vi "interfaz.vi"() -> ()   [LabVIEW 2020]
uses:
  proceso2.vi
  proceso1.vi
  proceso3.vi
  proceso5.vi
  proceso6.vi
  proceso4.vi
panel:
  in  "stop":bool
  out "TEMPERATURA  FINAL":dbl
  out "TEMPERATURA REFIRGERADOR":dbl
  out "caja 2":u8(slide) scale=0.0..100.0
  out "vent3":bool
  out "vent2":bool
  out "vent1":bool
  out "CONTADOR DE CAJAS":dbl
  out "sensor_caja":bool
  out "TEMPERATURA  INTERCAMBIADOR":dbl
  out "caja":u8(slide) scale=0.0..100.0
  out "sensor_inter":bool
  out "sensor_final":bool
  out "tuberia_5":u8(slide) scale=0.0..100.0
  out "tuberia_3":u8(slide) scale=0.0..100.0
  out "tuberia_6":u8(slide) scale=0.0..100.0
  out "tuberia_2":u8(slide) scale=0.0..100.0
  out "tuberia_4":u8(slide) scale=0.0..100.0
  out "tuberia_1":u8(slide) scale=0.0..100.0
  out "tanque_out":u8(slide) scale=0.0..100.0
  out "tanque in":u8(slide) scale=0.0..100.0
  out "sensor_ref":bool
  out "sensor bomba 1":bool
  out "sensor bomba dos":bool
  out "sensor_cal":bool
  # "SISTEMA DE PASTEURIZACION DE LECHE"
  # "TANQUE DE ENTRADA"
  # "TANQUE OUT"
  # "FINAL DE LINEA"
  # "DISTRIBUIDORA"
  # "REFRIGERADOR"
  # "INTERCAMBIADOR DE CALOR"
  # "BOMBA 1"
  # "CALDERA"
  # "BOMBA 2"
  # "PANEL"
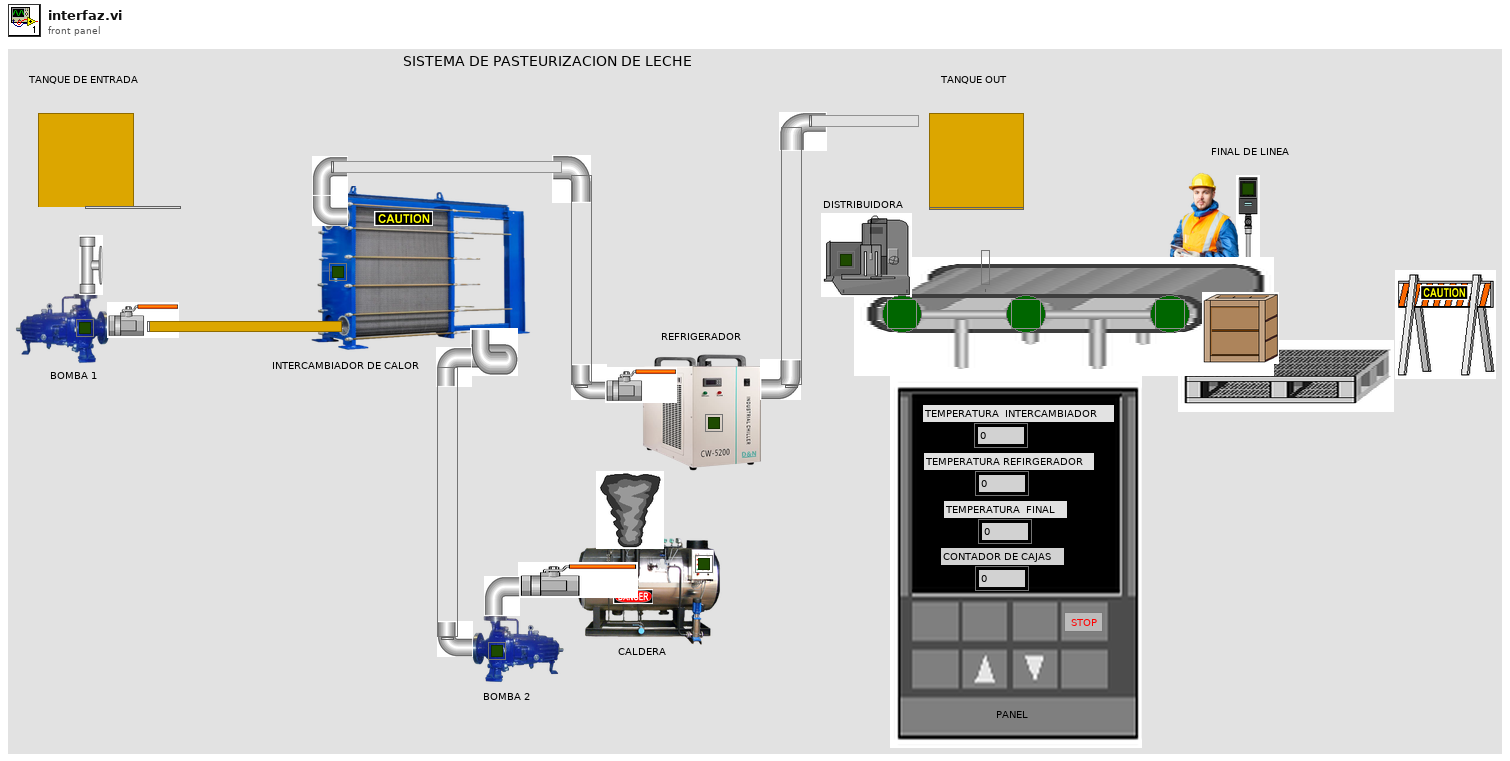
[diagram p1: front panel]
types:
  T1 = cluster{"final_linea":bool, "vent 1":bool, "vent 2":bool, "vent 3":bool, "mov caja horizontal":i32, "llenado caja":u8, "pos_inicial_horizontal":dbl, " pos_final_horizontal":dbl, "contador":dbl, "mov caja  vertical":i32, "pos_inicial_vertical":dbl, " pos_final_vertical":dbl}
  T2 = cluster{"sensor_caja":bool, "vent 1":bool, "vent 2":bool, "vent 3":bool, "pos_inicial":dbl, "pos_final":dbl, "mov_caja":i32}
  T3 = cluster{"sensor_refrigerador":bool, "temperatura":dbl, "tuberia 5":u8, "tuberia 6":u8}
  T4 = cluster{"sensor_bomba_1":bool, "tanque in":u8, " tuberia 1":u8}
  T5 = cluster{"sensor_intercambiador":bool, "sensor_caldera":bool, "sensor_bomba_2 ":bool, "tuberia 2":u8, "tuberia 3":u8, "tuberia 4":u8, "temperatura":dbl}
  T6 = cluster{"sensor_caja":bool, "vent 1":bool, "vent 2":bool, "vent 3":bool, "pos_inicial":dbl, "pos_final":dbl, "mov_caja 1":i32}
  T7 = cluster{"final_linea":bool, "vent 1":bool, "vent 2":bool, "vent 3":bool, "mov caja 2 horizontal":i32, "llenado caja 2":u8, "pos_inicial_horizontal":dbl, " pos_final_horizontal":dbl, "contador":dbl, "mov caja 2  vertical":i32, "pos_inicial_vertical":dbl, " pos_final_vertical":dbl}
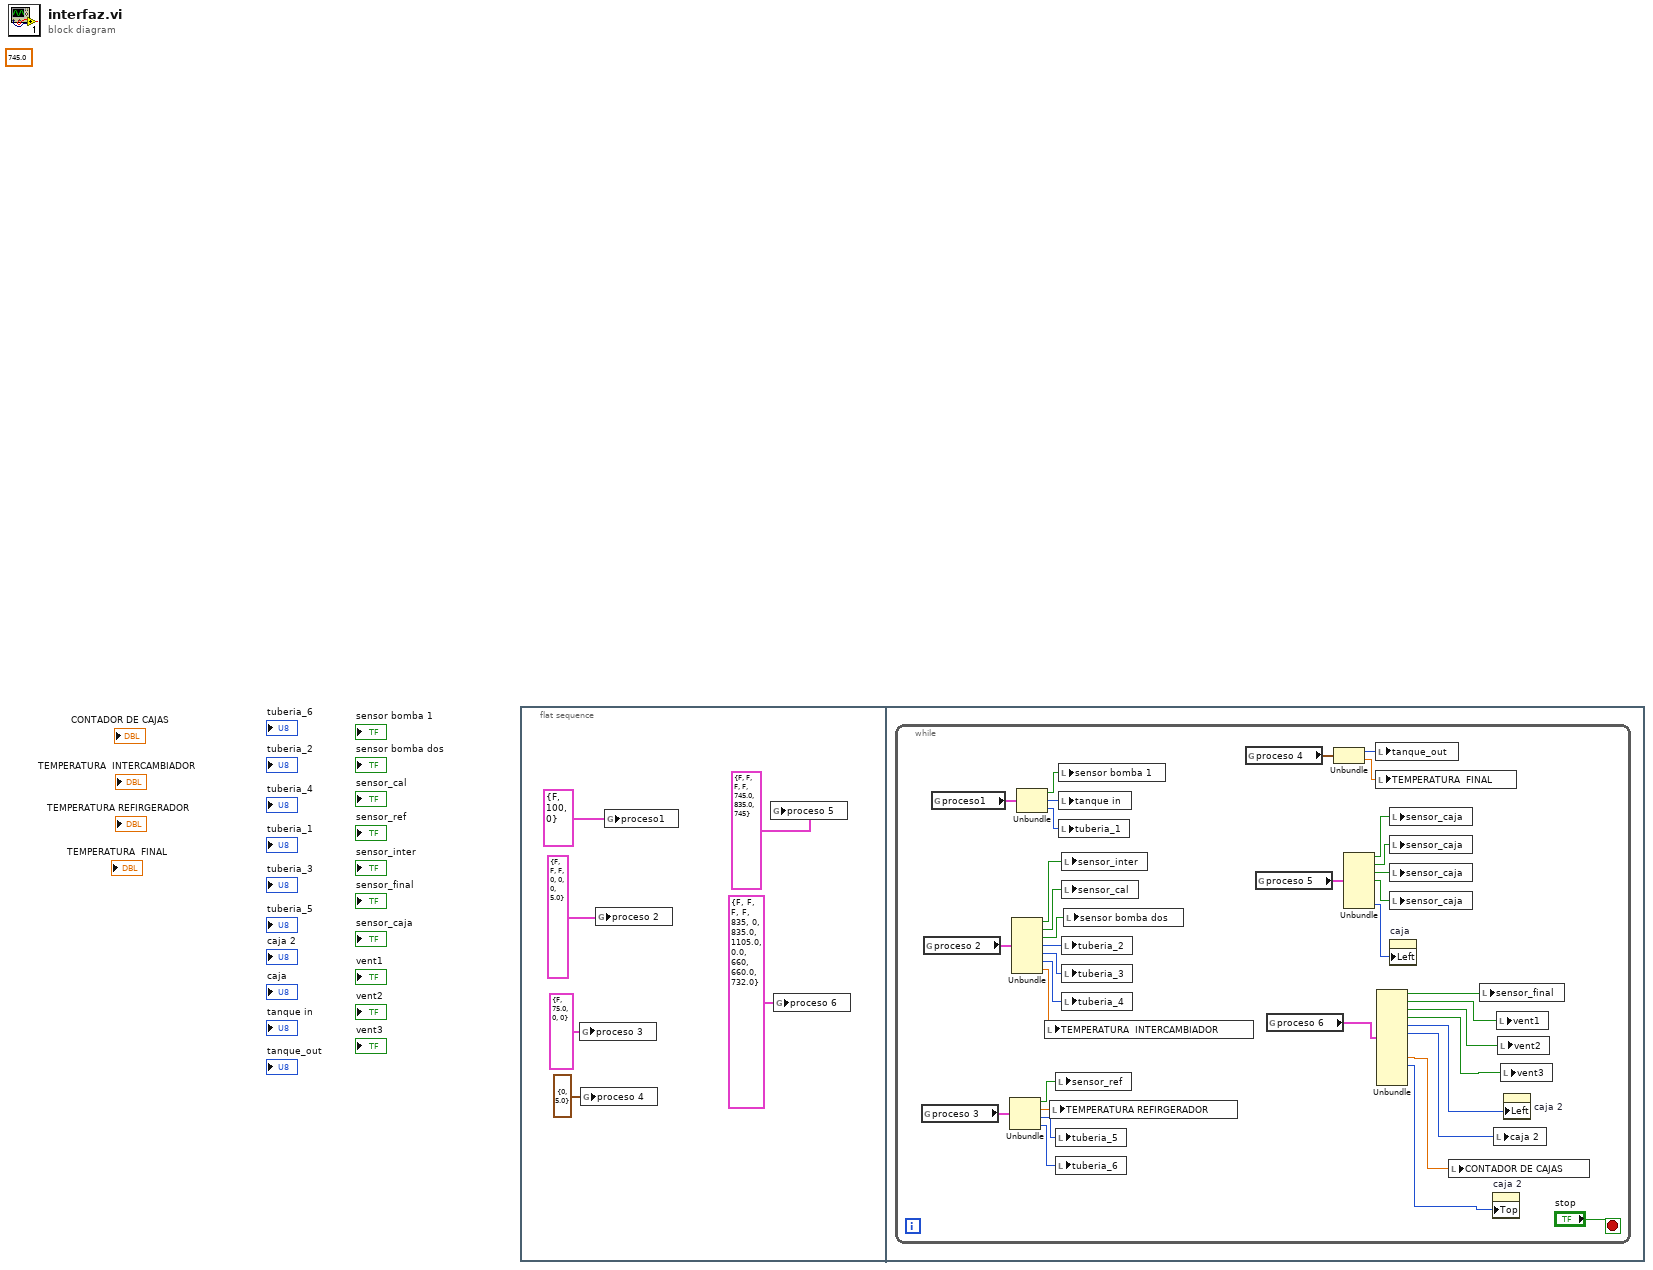
[diagram p0: block diagram]
diagram:
  (unwired) 745.0
  n1 = flat-sequence {
    frame #0 {
      n2 = global write "proceso3.vi" "proceso 3"(T3 {"sensor_refrigerador"=FALSE, "temperatura"=75.0, "tuberia 5"=0, "tuberia 6"=0} ("proceso 3")) -> ()
      n3 = global write "proceso4.vi" "proceso 4"(cluster{"tanque out":u8, "tempertura_final":dbl} {"tanque out"=0, "tempertura_final"=5.0} ("proceso 4")) -> ()
      n4 = global write "proceso2.vi" "proceso 2"(T5 {"sensor_intercambiador"=FALSE, "sensor_caldera"=FALSE, "sensor_bomba_2 "=FALSE, "tuberia 2"=0, "tuberia 3"=0, "tuberia 4"=0, "temperatura"=5.0} ("proceso 2")) -> ()
      n5 = global write "proceso1.vi" "proceso1"(T4 {"sensor_bomba_1"=FALSE, "tanque in"=100, " tuberia 1"=0} ("proceso1")) -> ()
      n6 = global write "proceso5.vi" "proceso 5"(T2 {"sensor_caja"=FALSE, "vent 1"=FALSE, "vent 2"=FALSE, "vent 3"=FALSE, "pos_inicial"=745.0, "pos_final"=835.0, "mov_caja"=745} ("proceso 5")) -> ()
      n7 = global write "proceso6.vi" "proceso 6"(T1 {"final_linea"=FALSE, "vent 1"=FALSE, "vent 2"=FALSE, "vent 3"=FALSE, "mov caja horizontal"=835, "llenado caja"=0, "pos_inicial_horizontal"=835.0, " pos_final_horizontal"=1105.0, "contador"=0.0, "mov caja  vertical"=660, "pos_inicial_vertical"=660.0, " pos_final_vertical"=732.0} ("proceso 6")) -> ()
    }
    frame #1 {
      n8 = while {
        stop <- "stop" stop-if-true
        n9 = global read "proceso3.vi" "proceso 3"() -> (w29:T3)
        n10 = global read "proceso2.vi" "proceso 2"() -> (w30:T5)
        n11 = global read "proceso1.vi" "proceso1"() -> (w38:T4)
        n12 = Unbundle(w29) -> ("sensor_refrigerador"=w28:bool, "temperatura"=w27:dbl, "tuberia 5"=w26:u8, "tuberia 6"=w25:u8)
        n13 = Unbundle(w30) -> ("sensor_intercambiador"=w35:bool, "sensor_caldera"=w36:bool, "sensor_bomba_2"=w37:bool, "tuberia 2"=w34:u8, "tuberia 3"=w33:u8, "tuberia 4"=w32:u8, "temperatura"=w31:dbl)
        n14 = Unbundle(w38) -> ("sensor_bomba_1"=w41:bool, "tanque in"=w39:u8, "tuberia 1"=w40:u8)
        n15 = local write "TEMPERATURA  INTERCAMBIADOR"(w31) -> ()
        n16 = local write "TEMPERATURA REFIRGERADOR"(w27) -> ()
        n17 = local write "sensor_ref"(w28) -> ()
        n18 = local write "tuberia_5"(w26) -> ()
        n19 = local write "tuberia_6"(w25) -> ()
        n20 = local write "sensor bomba 1"(w41) -> ()
        n21 = local write "tanque in"(w39) -> ()
        n22 = local write "tuberia_1"(w40) -> ()
        n23 = local write "sensor_inter"(w35) -> ()
        n24 = local write "sensor_cal"(w36) -> ()
        n25 = local write "tuberia_2"(w34) -> ()
        n26 = local write "tuberia_3"(w33) -> ()
        n27 = local write "tuberia_4"(w32) -> ()
        n28 = local write "sensor bomba dos"(w37) -> ()
        n29 = global read "proceso4.vi" "proceso 4"() -> (w24:cluster{"tanque out":u8, "tempertura_final":dbl})
        n30 = global read "proceso5.vi" "proceso 5"() -> (w22:T6)
        n31 = global read "proceso6.vi" "proceso 6"() -> (w16:T7)
        n32 = Unbundle(w24) -> ("tanque out"=w23:u8, "tempertura_final"=w7:dbl)
        n33 = Unbundle(w22) -> ("sensor_caja"=w21:bool, "vent 1"=w20:bool, "vent 2"=w19:bool, "vent 3"=w18:bool, "mov_caja 1"=w17:i32)  [unwired: 2 out]
        n34 = local write "tanque_out"(w23) -> ()
        n35 = local write "TEMPERATURA  FINAL"(w7) -> ()
        n36 = Unbundle(w16) -> ("final_linea"=w15:bool, "vent 1"=w14:bool, "vent 2"=w13:bool, "vent 3"=w12:bool, "mov caja 2 horizontal"=w9:i32, "llenado caja 2"=w11:u8, "contador"=w10:dbl, "mov caja 2  vertical"=w8:i32)  [unwired: 4 out]
        n37 = local write "sensor_caja"(w21) -> ()
        n38 = local write "sensor_caja"(w20) -> ()
        n39 = local write "sensor_caja"(w19) -> ()
        n40 = local write "sensor_caja"(w18) -> ()
        n41 = property on="caja" class="Slide (strict)"("Left"=w17) -> ()  [unwired: 2 in, 2 out]
        n42 = local write "CONTADOR DE CAJAS"(w10) -> ()
        n43 = local write "sensor_final"(w15) -> ()
        n44 = property on="caja 2" class="Slide (strict)"("Top"=w8) -> ()  [unwired: 2 in, 2 out]
        n45 = local write "caja 2"(w11) -> ()
        n46 = local write "vent1"(w14) -> ()
        n47 = local write "vent2"(w13) -> ()
        n48 = local write "vent3"(w12) -> ()
        n49 = property on="caja 2" class="Slide (strict)"("Left"=w9) -> ()  [unwired: 2 in, 2 out]
      }
    }
  }
